vi "SCLN_InitServers.vi"(2 "Config File Name":path, 3 "Server Names":string[](array[string]), 4 "Num of Servers":i32=1 min=1 max=7) -> (0 "error out":errorcluster)   [LabVIEW 2015]
uses:
  SCLN_NOTIF_Select.ctl
  SCLN_RW_Select.ctl
  SCLN_INT32_Select.ctl
panel:
  in  "error in (no error)":errorcluster
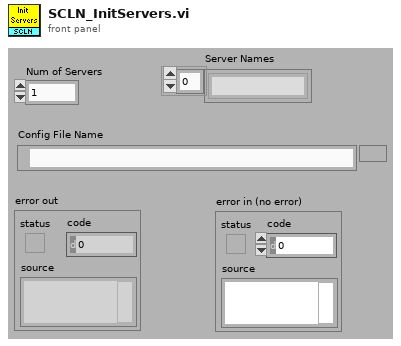
[diagram p1: front panel]
types:
  T1 = typedef "SCLN_INT32_Select.ctl" = enum16{"Max_Servers", "Max_Clients", "Total_Servers", "Total_Clients"}
  T2 = typedef "SCLN_RW_Select.ctl" = enum16{"Read", "Write"}
  T3 = typedef "SCLN_NOTIF_Select.ctl" = enum16{"Server1", "Server2", "Server3", "Server4", "Server5", "Server6", "Server7", "Client1", "Client2", "Client3", "Client4", "Client5", "Client6", "Client7", "Client8", "Client9", "Client10", "Shutdown", "Init_Ready"}
  T4 = typedef "SCLN_InfoClusterConfig.ctl" = cluster{"Section Name":string, "IP_Server":string, "IP_Client":string, "IP_Port":string}
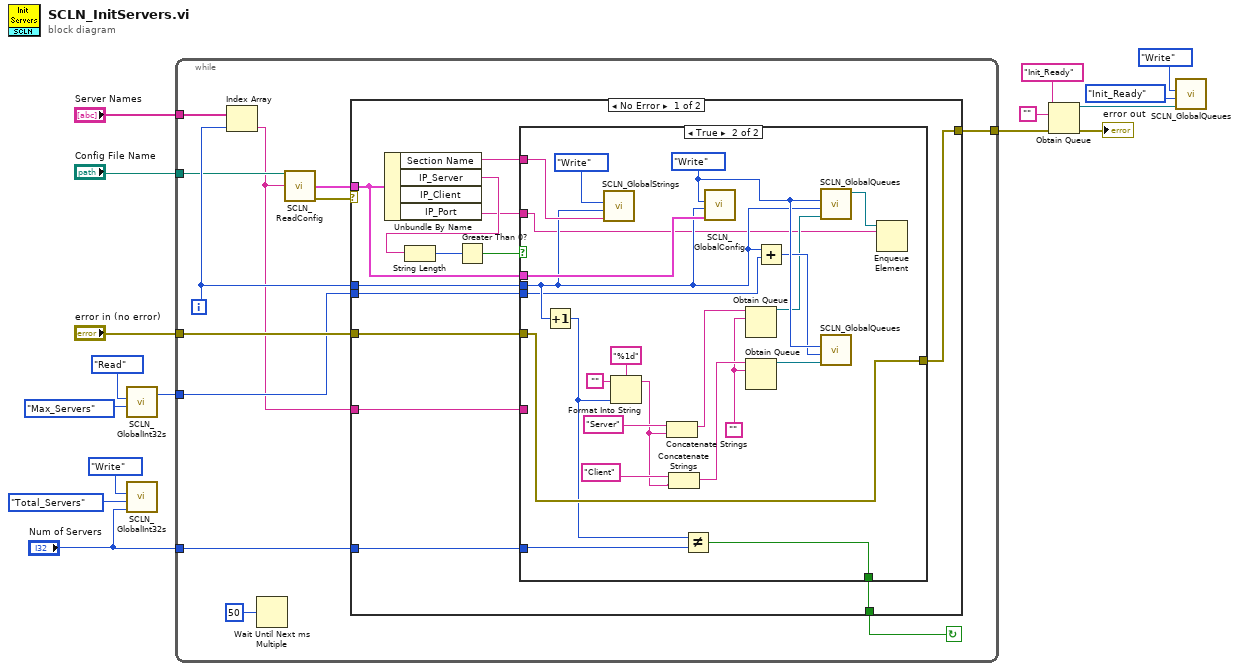
[diagram p0: block diagram]
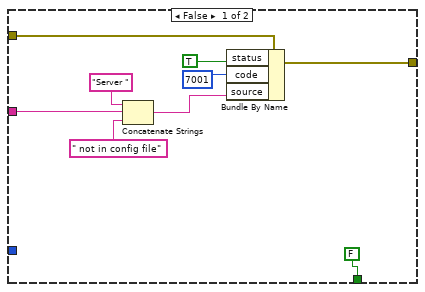
[diagram p2: hidden frame]
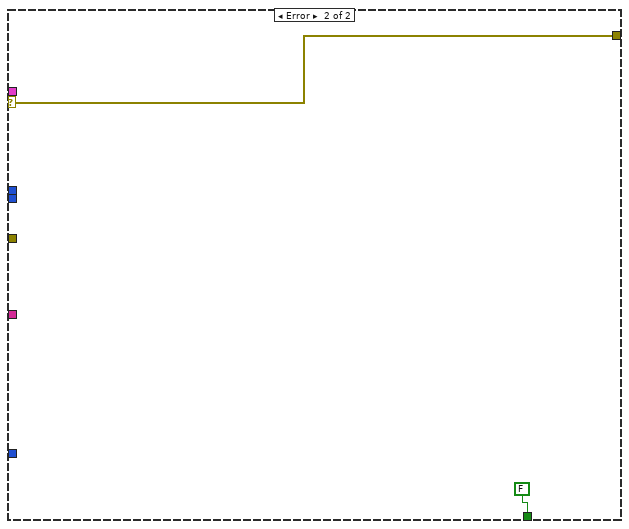
[diagram p3: hidden frame]
diagram:
  n1 = call "SCLN_GlobalInt32s.vi"("Element"=SCLN_INT32_Select."Max_Servers" ("GBL_INT32"), "Operation"=SCLN_RW_Select."Read" ("GBL_RW")) -> ("Read Value"=w6:i32)  [unwired: 2 in, 1 out]
  n2 = call "SCLN_GlobalInt32s.vi"("Write Value"="Num of Servers", "Element"=SCLN_INT32_Select."Total_Servers" ("GBL_INT32"), "Operation"=SCLN_RW_Select."Write" ("GBL_RW")) -> ()  [unwired: 1 in, 2 out]
  n3 = while {
    tunnel: [w26] -> w3
    tunnel: "error in (no error)" -> [w23]
    tunnel: "Num of Servers" -> [w22]
    tunnel: "Config File Name" -> [w21]
    tunnel: "Server Names" -> [w20]
    tunnel: w6 -> [w19]
    i -> [w24]
    stop <- w28 continue-if-true
    n4 = Index Array(array=w20, index=w24) -> (element=w18:string)
    n5 = Wait Until Next ms Multiple(millisecond multiple=50) -> ()  [unwired: 1 out]
    n6 = call "SCLN_ReadConfig.vi"("File Path"=w21, "Section Name"=w18) -> ("IP Info Connection"=w25:T4, "error out"=w27:errorcluster)  [unwired: 12 in]
    n7 = case shown="No Error" w27 {
      selector: w27 -> [_ w74]
      tunnel: [w35 FALSE] -> w28
      tunnel: [w33 w74] -> w26
      tunnel: w25 -> [w39 _]
      tunnel: w24 -> [w40 _]
      tunnel: w23 -> [w34 _]
      tunnel: w22 -> [w31 _]
      tunnel: w19 -> [w30 _]
      tunnel: w18 -> [w29 _]
      frame No Error {
        n8 = Unbundle By Name(w39) -> ("Section Name"=w41:string, "IP_Server"=w38:string, "IP_Port"=w32:string)  [unwired: 1 out]
        n9 = String Length(string=w38) -> (length=w37:i32)
        n10 = Greater Than 0?(x=w37) -> (x > 0?=w36:bool)
        n11 = case shown="True" w36 {
          tunnel: w41 -> [_ w72]
          tunnel: w40 -> [_ w63]
          tunnel: w39 -> [_ w71]
          tunnel: [FALSE w60] -> w35
          tunnel: w34 -> [w49 w62]
          tunnel: [w46 w62] -> w33
          tunnel: w32 -> [_ w52]
          tunnel: w31 -> [_ w59]
          tunnel: w30 -> [_ w58]
          tunnel: w29 -> [w44 _]
          frame False {
            n12 = Concatenate Strings("Server ", w44, " not in config file") -> (w42:string)
            n13 = Bundle By Name(cluster=w49, "status"=TRUE, "code"=7001, "source"=w42) -> (w46:errorcluster)
          }
          frame True {
            w51 = ""
            w65 = SCLN_RW_Select."Write" ("GBL_RW")
            n14 = Increment(x=w63) -> (x+1=w61:i32)
            n15 = call "SCLN_GlobalStrings.vi"("Write Value"=w72, "Element"=w63, "Operation"=SCLN_RW_Select."Write" ("GBL_RW")) -> ()  [unwired: 1 in, 2 out]
            n16 = Format Into String(format string="%1d", initial string="", w61) -> (resulting string=w66:string)  [unwired: 1 in, 1 out]
            n17 = Concatenate Strings("Server", w66) -> (w56:string)
            n18 = Concatenate Strings("Client", w66) -> (w57:string)
            n19 = Not Equal?(x=w61, y=w59) -> (x != y?=w60:bool)
            n20 = call "SCLN_GlobalConfig.vi"("Write Value"=w71, "Element"=w63, "Operation"=w65) -> ()  [unwired: 1 in, 2 out]
            n21 = Obtain Queue(name (unnamed)=w56, element data type=w51) -> (queue out=w55:refnum<queue>)  [unwired: 3 in, 2 out]
            n22 = Obtain Queue(name (unnamed)=w57, element data type=w51) -> (queue out=w54:refnum<queue>)  [unwired: 3 in, 2 out]
            n23 = Add(x=w63, y=w58) -> (x+y=w64:i32)
            n24 = call "SCLN_GlobalQueues.vi"("Write QueueID"=w55, "Element"=w63, "Operation"=w65) -> ("Read QueueID"=w53:refnum<queue>)  [unwired: 5 in, 1 out]
            n25 = call "SCLN_GlobalQueues.vi"("Write QueueID"=w54, "Element"=w64, "Operation"=w65) -> ()  [unwired: 5 in, 2 out]
            n26 = Enqueue Element(queue=w53, element=w52) -> ()  [unwired: 2 in, 3 out]
          }
        }
      }
      frame Error {
      }
    }
  }
  n27 = Obtain Queue(name (unnamed)="Init_Ready", element data type="", error in (no error)=w3) -> (queue out=w4:refnum<queue>, error out=→"error out":errorcluster)  [unwired: 2 in, 1 out]
  n28 = call "SCLN_GlobalQueues.vi"("Write QueueID"=w4, "Element"=SCLN_NOTIF_Select."Init_Ready" ("Dome String Ctrl"), "Operation"=SCLN_RW_Select."Write" ("GBL_RW")) -> ()  [unwired: 5 in, 2 out]
